vi "Start Long Running Process.vi"(6 "Promise":refnum<class "Promise.lvclass">, 8 "error in (no error)":errorcluster, 11 "Actor Example in":refnum<class "Actor Example.lvclass">) -> (0 "error out":errorcluster, 3 "Actor Example out":refnum<class "Actor Example.lvclass">)   [LabVIEW 2017, in "Actor Example.lvlib" / "Actor Example.lvclass"]
uses:
  Actor Example.lvclass
  C:/Program Files (x86)/National Instruments/LabVIEW 2017/vi.lib/ActorFramework/Actor/Actor.lvclass
  Promise Future/Promise/Promise.lvclass
  Long Running Process/Long Running Process.lvclass
  Actor Example.lvclass/Actor Example.ctl
  <vilib>/ActorFramework/Actor/Actor.lvclass
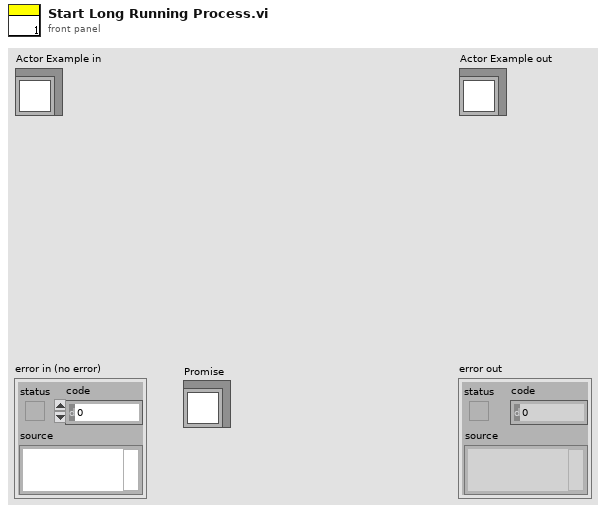
[diagram p1: front panel]
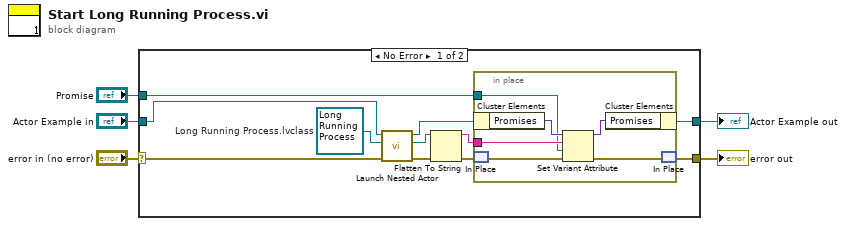
[diagram p0: block diagram]
diagram:
  n1 = case shown="No Error" "error in (no error)" {
    selector: "error in (no error)" -> [w7 w24]
    tunnel: [w10 w24] -> w4
    tunnel: [w9 w23] -> w2
    tunnel: "Actor Example in" -> [w16 w23]
    tunnel: "Promise" -> [w8 _]
    frame No Error {
      w6 = refnum<class "Long Running Process.lvclass"> refnum  # Long Running Process.lvclass
      n2 = call <vilib>:"Launch Nested Actor.vi"("error in (no error)"=w7, "Nested Actor"=w6, "Caller Actor in"=w16) -> ("error out"=w12:errorcluster, "Nested Actor's Enqueuer"=w14:refnum<class "Message Enqueuer.lvclass">, "Caller Actor out"=w15:refnum<class "Actor Example.lvclass">)  [unwired: 6 in]
      n3 = Flatten To String(anything=w14, error in (no error)=w12) -> (data string=w13:string, error out=w11:errorcluster)  [unwired: 2 in, 1 out]
      n4 = in-place {
        in-place-border: w13 -> [w20]
        in-place-border: w8 -> [w19]
        n5 = in-place-cluster #1(w15) -> ("Promises"=w22:variant)
        n6 = in-place-match #2(w11) -> (w18:errorcluster)
        n7 = Set Variant Attribute(Variant=w22, name=w20, value=w19, error in=w18) -> (Variant out=w21:variant, error out=w17:errorcluster)  [unwired: 1 out]
        n8 = in-place-cluster #1("Promises"=w21) -> (w9:refnum<class "Actor Example.lvclass">)
        n9 = in-place-match #2(w17) -> (w10:errorcluster)
      }
    }
    frame Error {
    }
  }
  "error out" <- w4
  "Actor Example out" <- w2
